vi "PCO_Description2.vi"() -> (0 "PCO_Description2":T1 {"dwModulateCapsDESC2" format="%x"}, 1 "PCO_Description2_Raw":T2, 2 "Length":u16, 3 "Raw_Length":u16)   [LabVIEW 2019, in "SDK.lvlib" / "Structures.lvlib"]
doc: "Use this template to build a VI to use as a subVI."
uses:
  Structures.lvlib
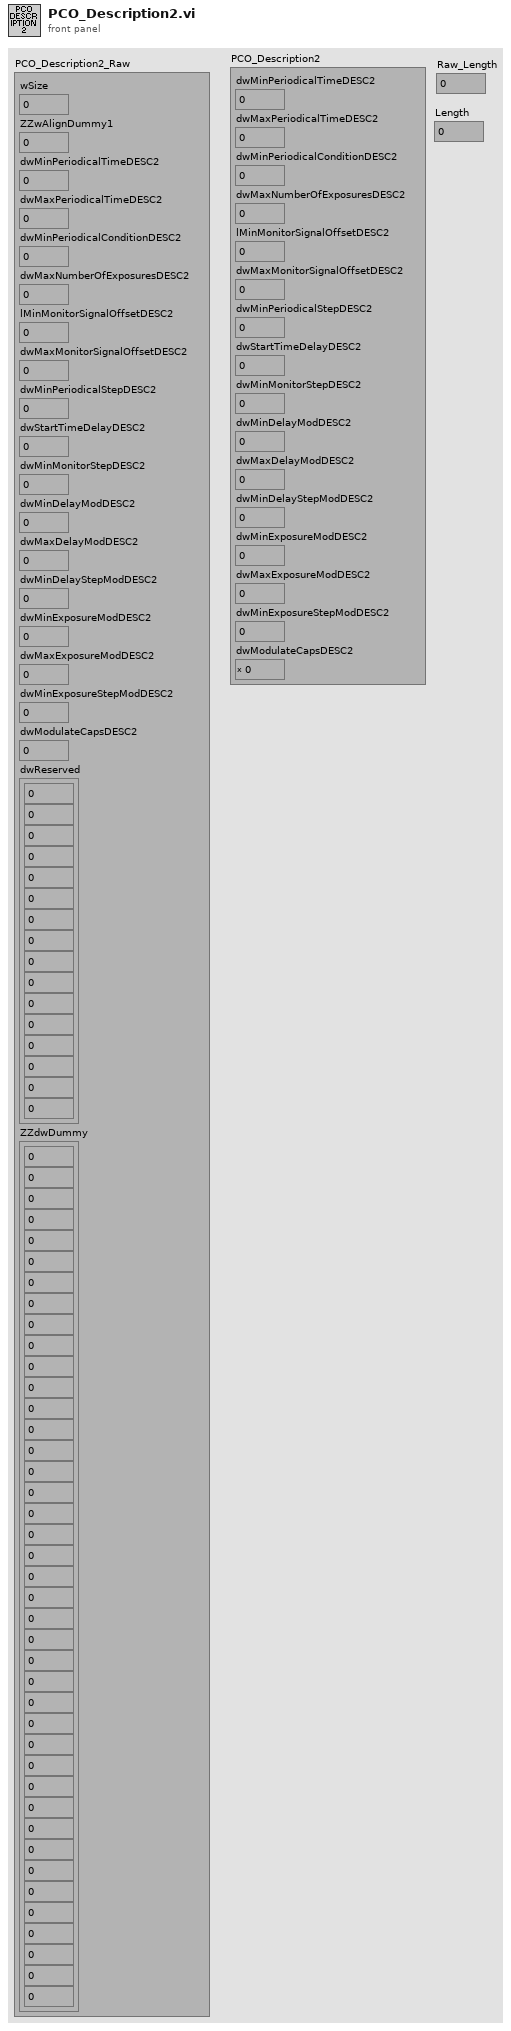
[diagram p1: front panel]
types:
  T1 = cluster{"dwMinPeriodicalTimeDESC2":u32, "dwMaxPeriodicalTimeDESC2":u32, "dwMinPeriodicalConditionDESC2":u32, "dwMaxNumberOfExposuresDESC2":u32, "lMinMonitorSignalOffsetDESC2":i32, "dwMaxMonitorSignalOffsetDESC2":u32, "dwMinPeriodicalStepDESC2":u32, "dwStartTimeDelayDESC2":u32, "dwMinMonitorStepDESC2":u32, "dwMinDelayModDESC2":u32, "dwMaxDelayModDESC2":u32, "dwMinDelayStepModDESC2":u32, "dwMinExposureModDESC2":u32, "dwMaxExposureModDESC2":u32, "dwMinExposureStepModDESC2":u32, "dwModulateCapsDESC2":u32}
  T2 = cluster{"wSize":u16, "ZZwAlignDummy1":u16, "dwMinPeriodicalTimeDESC2":u32, "dwMaxPeriodicalTimeDESC2":u32, "dwMinPeriodicalConditionDESC2":u32, "dwMaxNumberOfExposuresDESC2":u32, "lMinMonitorSignalOffsetDESC2":i32, "dwMaxMonitorSignalOffsetDESC2":u32, "dwMinPeriodicalStepDESC2":u32, "dwStartTimeDelayDESC2":u32, "dwMinMonitorStepDESC2":u32, "dwMinDelayModDESC2":u32, "dwMaxDelayModDESC2":u32, "dwMinDelayStepModDESC2":u32, "dwMinExposureModDESC2":u32, "dwMaxExposureModDESC2":u32, "dwMinExposureStepModDESC2":u32, "dwModulateCapsDESC2":u32, "dwReserved":cluster{u32, u32, u32, u32, u32, u32, u32, u32, u32, u32, u32, u32, u32, u32, u32, u32}, "ZZdwDummy":cluster{u32, u32, u32, u32, u32, u32, u32, u32, u32, u32, u32, u32, u32, u32, u32, u32, u32, u32, u32, u32, u32, u32, u32, u32, u32, u32, u32, u32, u32, u32, u32, u32, u32, u32, u32, u32, u32, u32, u32, u32, u32}}
  T3 = cluster{u32, u32, u32, u32, u32, u32, u32, u32, u32, u32, u32, u32, u32, u32, u32, u32, u32, u32, u32, u32, u32, u32, u32, u32, u32, u32, u32, u32, u32, u32, u32, u32, u32, u32, u32, u32, u32, u32, u32, u32, u32}
  T4 = cluster{u32, u32, u32, u32, u32, u32, u32, u32, u32, u32, u32, u32, u32, u32, u32, u32}
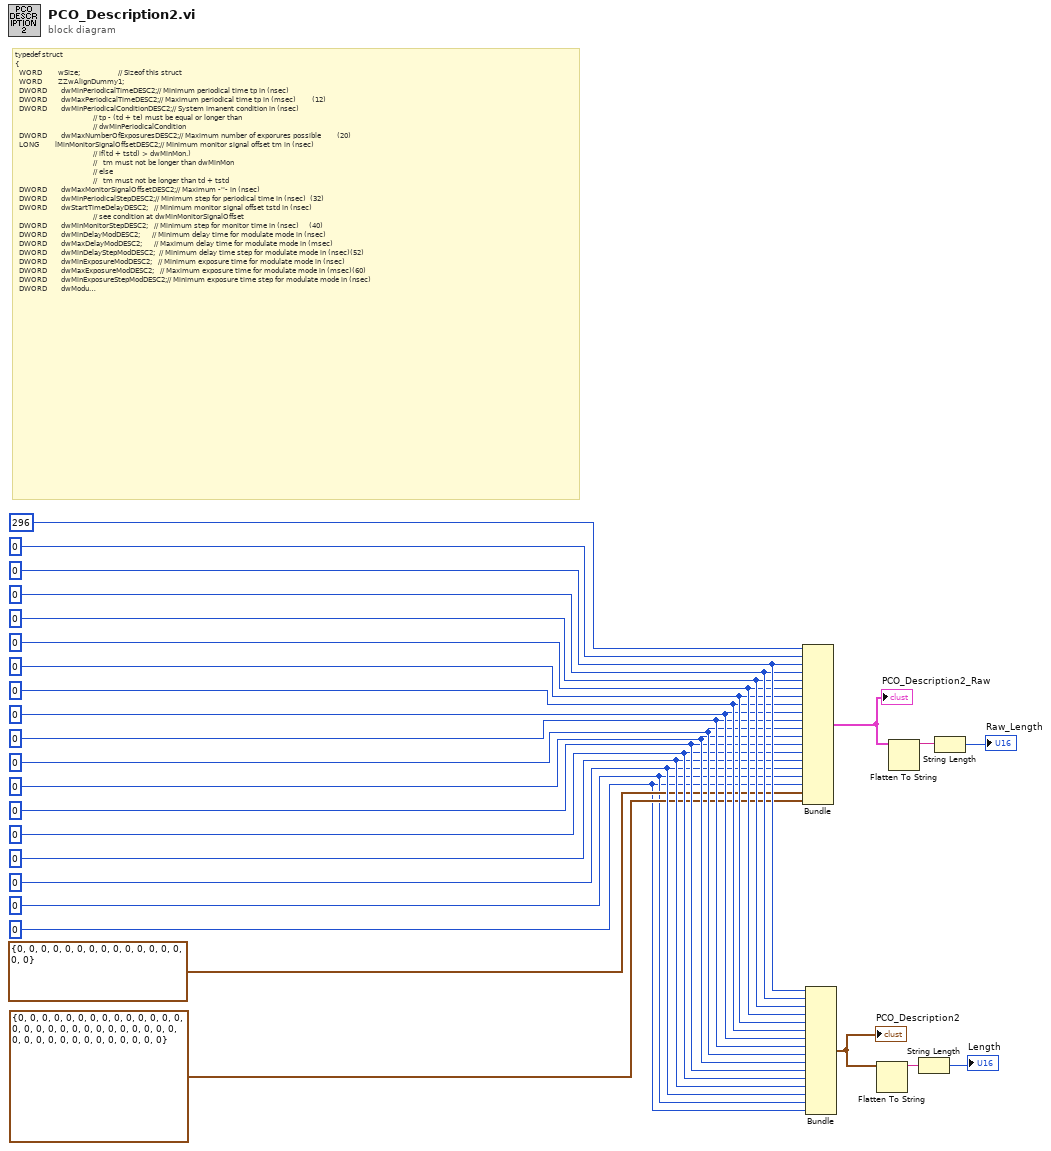
[diagram p0: block diagram]
diagram:
  w1 = u32 0 ("dwModulateCapsDESC2")
  w2 = u32 0 ("dwMinExposureStepModDESC2")
  w6 = u32 0 ("dwMaxExposureModDESC2")
  w7 = u32 0 ("dwMinExposureModDESC2")
  w8 = u32 0 ("dwMinDelayStepModDESC2")
  w9 = u32 0 ("dwMaxDelayModDESC2")
  w10 = u32 0 ("dwMinDelayModDESC2")
  w11 = u32 0 ("dwMinMonitorStepDESC2")
  w12 = u32 0 ("dwStartTimeDelayDESC2")
  w13 = u32 0 ("dwMinPeriodicalStepDESC2")
  w14 = u32 0 ("dwMaxMonitorSignalOffsetDESC2")
  w15 = 0 ("lMinMonitorSignalOffsetDESC2")
  w16 = u32 0 ("dwMaxNumberOfExposuresDESC2")
  w17 = u32 0 ("dwMinPeriodicalConditionDESC2")
  w18 = u32 0 ("dwMaxPeriodicalTimeDESC2")
  w19 = u32 0 ("dwMinPeriodicalTimeDESC2")
  # "typedef struct\n{\n  WORD        wSize;                   // Sizeof this struct\n  WORD        ZZwAlignDummy1;\n  DWORD       dwMinPeriodicalTimeDESC2;// Minimum periodical time tp in (nsec)\n  DWORD       dwMaxPeriodicalTimeDESC2;// Maximum periodical time tp in (msec)        (12)\n  DWORD       dwMinPeriodicalConditionDESC2;// System imanent condition in (nsec)\n                                       // tp - (td + te) must be equal or longer than\n                                       // dwMinPeriodicalCondition\n  DWORD       dwMaxNumberOfExposuresDESC2;// Maximum number of exporures possible        (20)\n  LONG        lMinMonitorSignalOffsetDESC2;// Minimum monitor signal offset tm in (nsec)\n                                       // if(td + tstd) > dwMinMon.)\n                                       //   tm must not be longer than dwMinMon\n                                       // else\n                                       //   tm must not be longer than td + tstd\n  DWORD       dwMaxMonitorSignalOffsetDESC2;// Maximum -''- in (nsec)                      \n  DWORD       dwMinPeriodicalStepDESC2;// Minimum step for periodical time in (nsec)  (32)\n  DWORD       dwStartTimeDelayDESC2;   // Minimum monitor signal offset tstd in (nsec)\n                                       // see condition at dwMinMonitorSignalOffset\n  DWORD       dwMinMonitorStepDESC2;   // Minimum step for monitor time in (nsec)     (40)\n  DWORD       dwMinDelayModDESC2;      // Minimum delay time for modulate mode in (nsec)\n  DWORD       dwMaxDelayModDESC2;      // Maximum delay time for modulate mode in (msec)\n  DWORD       dwMinDelayStepModDESC2;  // Minimum delay time step for modulate mode in (nsec)(52)\n  DWORD       dwMinExposureModDESC2;   // Minimum exposure time for modulate mode in (nsec)\n  DWORD       dwMaxExposureModDESC2;   // Maximum exposure time for modulate mode in (msec)(60)\n  DWORD       dwMinExposureStepModDESC2;// Minimum exposure time step for modulate mode in (nsec)\n  DWORD       dwModulateCapsDESC2;     // Modulate capabilities descriptor\n  DWORD       dwReserved[16];                                                         //(132)\n  DWORD       ZZdwDummy[41];                                                          // 296\n} PCO_Description2;"
  n1 = Bundle("wSize"=u16 296, "ZZwAlignDummy1"=u16 0, "dwMinPeriodicalTimeDESC2"=w19, "dwMaxPeriodicalTimeDESC2"=w18, "dwMinPeriodicalConditionDESC2"=w17, "dwMaxNumberOfExposuresDESC2"=w16, "lMinMonitorSignalOffsetDESC2"=w15, "dwMaxMonitorSignalOffsetDESC2"=w14, "dwMinPeriodicalStepDESC2"=w13, "dwStartTimeDelayDESC2"=w12, "dwMinMonitorStepDESC2"=w11, "dwMinDelayModDESC2"=w10, "dwMaxDelayModDESC2"=w9, "dwMinDelayStepModDESC2"=w8, "dwMinExposureModDESC2"=w7, "dwMaxExposureModDESC2"=w6, "dwMinExposureStepModDESC2"=w2, "dwModulateCapsDESC2"=w1, "dwReserved"=T4 {0, 0, 0, 0, 0, 0, 0, 0, 0, 0, 0, 0, 0, 0, 0, 0}, "ZZdwDummy"=T3 {0, 0, 0, 0, 0, 0, 0, 0, 0, 0, 0, 0, 0, 0, 0, 0, 0, 0, 0, 0, 0, 0, 0, 0, 0, 0, 0, 0, 0, 0, 0, 0, 0, 0, 0, 0, 0, 0, 0, 0, 0}) -> (w5:T2)  [unwired: 1 in]
  "PCO_Description2_Raw" <- w5
  n2 = Bundle("dwMinPeriodicalTimeDESC2"=w19, "dwMaxPeriodicalTimeDESC2"=w18, "dwMinPeriodicalConditionDESC2"=w17, "dwMaxNumberOfExposuresDESC2"=w16, "lMinMonitorSignalOffsetDESC2"=w15, "dwMaxMonitorSignalOffsetDESC2"=w14, "dwMinPeriodicalStepDESC2"=w13, "dwStartTimeDelayDESC2"=w12, "dwMinMonitorStepDESC2"=w11, "dwMinDelayModDESC2"=w10, "dwMaxDelayModDESC2"=w9, "dwMinDelayStepModDESC2"=w8, "dwMinExposureModDESC2"=w7, "dwMaxExposureModDESC2"=w6, "dwMinExposureStepModDESC2"=w2, "dwModulateCapsDESC2"=w1) -> (w26:T1)  [unwired: 1 in]
  "PCO_Description2" <- w26
  n3 = Flatten To String(anything=w26) -> (data string=w25:string)  [unwired: 3 in, 2 out]
  n4 = Flatten To String(anything=w5) -> (data string=w24:string)  [unwired: 3 in, 2 out]
  n5 = String Length(string=w25) -> (length=→"Length":i32)
  n6 = String Length(string=w24) -> (length=→"Raw_Length":i32)
